vi "Translation2d_RotateBy.vi"(9 "other Rotation":T1 {"SIN" format="%13.4f"; "COS" format="%13.4f"; "VALUE" format="%13.4f"}, 11 "In Translation":T2 {"Y" format="%14.3f"; "X" format="%14.3f"}) -> (3 "Out Translation":T2 {"Y" format="%14.3f"; "X" format="%14.3f"})   [LabVIEW 2019, in "Trajectory_Library.lvlib"]
doc: "Applies a rotation to the translation in 2d space.\n\nThis multiplies the translation vector by a counterclockwise rotation matrix of the given angle.\n [x_new] [other.cos, -other.sin][x]\n [y_new] = [other.sin, other.cos][y]\n \nFor example, rotating a Translation2d of {2, 0} by 90 degrees will return a Translation2d of {0, 2}.\n\nParameters:\n - In Translation - This data structure\n - Other Rotation - The rotation to rotate the translation by. \n\nReturns:\n - Out Translation - The resulting Translation data structure"
uses:
  Trajectory_Library.lvlib
  TRANSLATION2D.ctl
  ROTATION2D.ctl
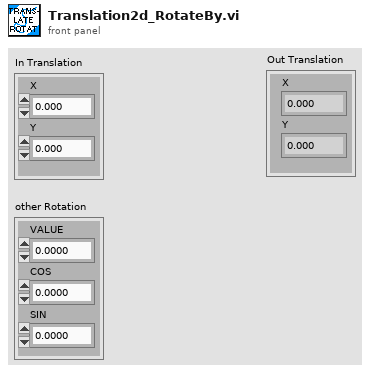
[diagram p1: front panel]
types:
  T1 = typedef "Trajectory_Library.lvlib/ROTATION2D.ctl" = cluster{"VALUE":dbl, "COS":dbl, "SIN":dbl}
  T2 = typedef "Trajectory_Library.lvlib/TRANSLATION2D.ctl" = cluster{"X":dbl, "Y":dbl}
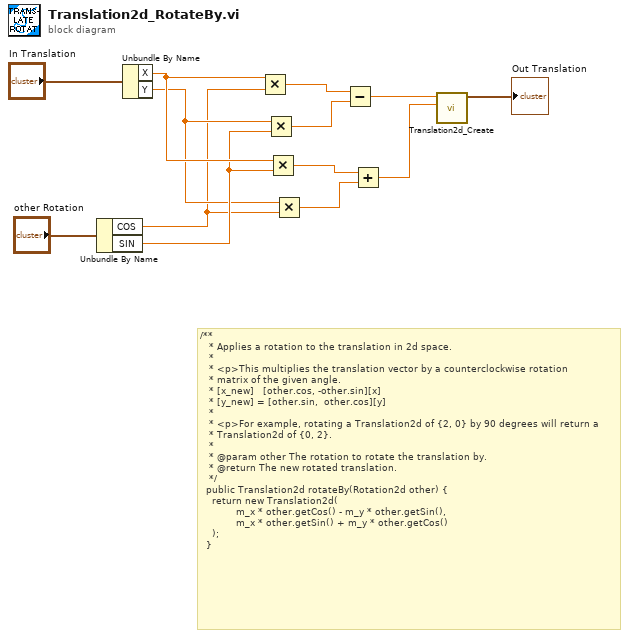
[diagram p0: block diagram]
diagram:
  # "/**\n   * Applies a rotation to the translation in 2d space.\n   *\n   * <p>This multiplies the translation vector by a counterclockwise rotation\n   * matrix of the given angle.\n   * [x_new]   [other.cos, -other.sin][x]\n   * [y_new] = [other.sin,  other.cos][y]\n   *\n   * <p>For example, rotating a Translation2d of {2, 0} by 90 degrees will return a\n   * Translation2d of {0, 2}.\n   *\n   * @param other The rotation to rotate the translation by.\n   * @return The new rotated translation.\n   */\n  public Translation2d rotateBy(Rotation2d other) {\n    return new Translation2d(\n            m_x * other.getCos() - m_y * other.getSin(),\n            m_x * other.getSin() + m_y * other.getCos()\n    );\n  }"
  n1 = Unbundle By Name("other Rotation") -> ("COS"=w4:dbl, "SIN"=w6:dbl)
  n2 = Unbundle By Name("In Translation") -> ("X"=w7:dbl, "Y"=w5:dbl)
  n3 = Multiply(x=w7, y=w4) -> (x*y=w11:dbl)
  n4 = Multiply(x=w5, y=w6) -> (x*y=w10:dbl)
  n5 = Multiply(x=w7, y=w6) -> (x*y=w9:dbl)
  n6 = Multiply(x=w5, y=w4) -> (x*y=w8:dbl)
  n7 = Subtract(x=w11, y=w10) -> (x-y=w2:dbl)
  n8 = Add(x=w9, y=w8) -> (x+y=w1:dbl)
  n9 = call "Translation2d_Create.vi"("Y"=w1, "X"=w2) -> ("TRANSLATION"=→"Out Translation":T2)  [unwired: 9 in]
